vi "test TCX read (installed 71).vi"() -> ()   [LabVIEW 2011] (continued)
armin.com/xmlschemas/ActivityExtension/v2\"><Watts>297</Watts></TPX></Extensions></Trackpoint><Trackpoint><Time>2008-03-03T13:51:13Z</Time><Position><LatitudeDegrees>35.881028</LatitudeDegrees><LongitudeDegrees>-78.947664</LongitudeDegrees></Position><AltitudeMeters>84.733</AltitudeMeters><DistanceMeters>1639.767</DistanceMeters><Cadence>88</Cadence><Extensions><TPX xmlns=\"http://www.garmin.com/xmlschemas/ActivityExtension/v2\"><Watts>240</Watts></TPX></Extensions></Trackpoint><Trackpoint><Time>2008-03-03T13:51:14Z</Time><Position><LatitudeDegrees>35.880933</LatitudeDegrees><LongitudeDegrees>-78.947691</LongitudeDegrees></Position><AltitudeMeters>84.733</AltitudeMeters><DistanceMeters>1650.482</DistanceMeters><Cadence>88</Cadence><Extensions><TPX xmlns=\"http://www.garmin.com/xmlschemas/ActivityExtension/v2\"><Watts>161</Watts></TPX></Extensions></Trackpoint><Trackpoint><Time>2008-03-03T13:51:15Z</Time><Position><LatitudeDegrees>35.880839</LatitudeDegrees><LongitudeDegrees>-78.947718</LongitudeDegrees></Position><AltitudeMeters>84.733</AltitudeMeters><DistanceMeters>1661.201</DistanceMeters><Cadence>87</Cadence><Extensions><TPX xmlns=\"http://www.garmin.com/xmlschemas/ActivityExtension/v2\"><Watts>138</Watts></TPX></Extensions></Trackpoint><Trackpoint><Time>2008-03-03T13:51:16Z</Time><Position><LatitudeDegrees>35.880745</LatitudeDegrees><LongitudeDegrees>-78.947745</LongitudeDegrees></Position><AltitudeMeters>84.253</AltitudeMeters><DistanceMeters>1671.990</DistanceMeters><Cadence>88</Cadence><Extensions><TPX xmlns=\"http://www.garmin.com/xmlschemas/ActivityExtension/v2\"><Watts>130</Watts></TPX></Extensions></Trackpoint><Trackpoint><Time>2008-03-03T13:51:17Z</Time><Position><LatitudeDegrees>35.880651</LatitudeDegrees><LongitudeDegrees>-78.947772</LongitudeDegrees></Position><AltitudeMeters>84.253</AltitudeMeters><DistanceMeters>1682.650</DistanceMeters><Cadence>88</Cadence><Extensions><TPX xmlns=\"http://www.garmin.com/xmlschemas/ActivityExtension/v2\"><Watts>130</Watts></TPX></Extensions></Trackpoint><Trackpoint><Time>2008-03-03T13:51:18Z</Time><Position><LatitudeDegrees>35.880555</LatitudeDegrees><LongitudeDegrees>-78.947798</LongitudeDegrees></Position><AltitudeMeters>83.772</AltitudeMeters><DistanceMeters>1693.542</DistanceMeters><Cadence>89</Cadence><Extensions><TPX xmlns=\"http://www.garmin.com/xmlschemas/ActivityExtension/v2\"><Watts>138</Watts></TPX></Extensions></Trackpoint><Trackpoint><Time>2008-03-03T13:51:19Z</Time><Position><LatitudeDegrees>35.880459</LatitudeDegrees><LongitudeDegrees>-78.947824</LongitudeDegrees></Position><AltitudeMeters>83.772</AltitudeMeters><DistanceMeters>1704.492</DistanceMeters><Cadence>90</Cadence><Extensions><TPX xmlns=\"http://www.garmin.com/xmlschemas/ActivityExtension/v2\"><Watts>159</Watts></TPX></Extensions></Trackpoint><Trackpoint><Time>2008-03-03T13:51:20Z</Time><Position><LatitudeDegrees>35.880357</LatitudeDegrees><LongitudeDegrees>-78.947852</LongitudeDegrees></Position><AltitudeMeters>83.291</AltitudeMeters><DistanceMeters>1716.066</DistanceMeters><Cadence>90</Cadence><Extensions><TPX xmlns=\"http://www.garmin.com/xmlschemas/ActivityExtension/v2\"><Watts>168</Watts></TPX></Extensions></Trackpoint><Trackpoint><Time>2008-03-03T13:51:21Z</Time><Position><LatitudeDegrees>35.880258</LatitudeDegrees><LongitudeDegrees>-78.947880</LongitudeDegrees></Position><AltitudeMeters>82.811</AltitudeMeters><DistanceMeters>1727.394</DistanceMeters><Cadence>91</Cadence><Extensions><TPX xmlns=\"http://www.garmin.com/xmlschemas/ActivityExtension/v2\"><Watts>169</Watts></TPX></Extensions></Trackpoint><Trackpoint><Time>2008-03-03T13:51:22Z</Time><Position><LatitudeDegrees>35.880159</LatitudeDegrees><LongitudeDegrees>-78.947909</LongitudeDegrees></Position><AltitudeMeters>83.291</AltitudeMeters><DistanceMeters>1738.638</DistanceMeters><Cadence>90</Cadence><Extensions><TPX xmlns=\"http://www.garmin.com/xmlschemas/ActivityExtension/v2\"><Watts>163</Watts></TPX></Extensions></Trackpoint><Trackpoint><Time>2008-03-03T13:51:23Z</Time><Position><LatitudeDegrees>35.880061</LatitudeDegrees><LongitudeDegrees>-78.947936</LongitudeDegrees></Position><AltitudeMeters>82.811</AltitudeMeters><DistanceMeters>1749.873</DistanceMeters><Cadence>85</Cadence><Extensions><TPX xmlns=\"http://www.garmin.com/xmlschemas/ActivityExtension/v2\"><Watts>162</Watts></TPX></Extensions></Trackpoint><Trackpoint><Time>2008-03-03T13:51:24Z</Time><Position><LatitudeDegrees>35.879962</LatitudeDegrees><LongitudeDegrees>-78.947964</LongitudeDegrees></Position><AltitudeMeters>82.811</AltitudeMeters><DistanceMeters>1761.036</DistanceMeters><Cadence>85</Cadence><Extensions><TPX xmlns=\"http://www.garmin.com/xmlschemas/ActivityExtension/v2\"><Watts>162</Watts></TPX></Extensions></Trackpoint><Trackpoint><Time>2008-03-03T13:51:25Z</Time><Position><LatitudeDegrees>35.879864</LatitudeDegrees><LongitudeDegrees>-78.947991</LongitudeDegrees></Position><AltitudeMeters>82.330</AltitudeMeters><DistanceMeters>1772.261</DistanceMeters><Cadence>87</Cadence><Extensions><TPX xmlns=\"http://www.garmin.com/xmlschemas/ActivityExtension/v2\"><Watts>298</Watts></TPX></Extensions></Trackpoint><Trackpoint><Time>2008-03-03T13:51:26Z</Time><Position><LatitudeDegrees>35.879765</LatitudeDegrees><LongitudeDegrees>-78.948017</LongitudeDegrees></Position><AltitudeMeters>82.330</AltitudeMeters><DistanceMeters>1783.429</DistanceMeters><Cadence>87</Cadence><Extensions><TPX xmlns=\"http://www.garmin.com/xmlschemas/ActivityExtension/v2\"><Watts>301</Watts></TPX></Extensions></Trackpoint><Trackpoint><Time>2008-03-03T13:51:27Z</Time><Position><LatitudeDegrees>35.879669</LatitudeDegrees><LongitudeDegrees>-78.948046</LongitudeDegrees></Position><AltitudeMeters>81.849</AltitudeMeters><DistanceMeters>1794.441</DistanceMeters><Cadence>87</Cadence><Extensions><TPX xmlns=\"http://www.garmin.com/xmlschemas/ActivityExtension/v2\"><Watts>261</Watts></TPX></Extensions></Trackpoint><Trackpoint><Time>2008-03-03T13:51:28Z</Time><Position><LatitudeDegrees>35.879570</LatitudeDegrees><LongitudeDegrees>-78.948074</LongitudeDegrees></Position><AltitudeMeters>81.849</AltitudeMeters><DistanceMeters>1805.737</DistanceMeters><Cadence>88</Cadence><Extensions><TPX xmlns=\"http://www.garmin.com/xmlschemas/ActivityExtension/v2\"><Watts>224</Watts></TPX></Extensions></Trackpoint><Trackpoint><Time>2008-03-03T13:51:29Z</Time><Position><LatitudeDegrees>35.879469</LatitudeDegrees><LongitudeDegrees>-78.948102</LongitudeDegrees></Position><AltitudeMeters>81.369</AltitudeMeters><DistanceMeters>1817.204</DistanceMeters><Cadence>88</Cadence><Extensions><TPX xmlns=\"http://www.garmin.com/xmlschemas/ActivityExtension/v2\"><Watts>225</Watts></TPX></Extensions></Trackpoint><Trackpoint><Time>2008-03-03T13:51:30Z</Time><Position><LatitudeDegrees>35.879367</LatitudeDegrees><LongitudeDegrees>-78.948129</LongitudeDegrees></Position><AltitudeMeters>81.369</AltitudeMeters><DistanceMeters>1828.736</DistanceMeters><Cadence>86</Cadence><Extensions><TPX xmlns=\"http://www.garmin.com/xmlschemas/ActivityExtension/v2\"><Watts>204</Watts></TPX></Extensions></Trackpoint><Trackpoint><Time>2008-03-03T13:51:31Z</Time><Position><LatitudeDegrees>35.879267</LatitudeDegrees><LongitudeDegrees>-78.948157</LongitudeDegrees></Position><AltitudeMeters>81.369</AltitudeMeters><DistanceMeters>1840.158</DistanceMeters><Cadence>87</Cadence><Extensions><TPX xmlns=\"http://www.garmin.com/xmlschemas/ActivityExtension/v2\"><Watts>241</Watts></TPX></Extensions></Trackpoint><Trackpoint><Time>2008-03-03T13:51:32Z</Time><Position><LatitudeDegrees>35.879166</LatitudeDegrees><LongitudeDegrees>-78.948183</LongitudeDegrees></Position><AltitudeMeters>81.369</AltitudeMeters><DistanceMeters>1851.623</DistanceMeters><Cadence>87</Cadence><Extensions><TPX xmlns=\"http://www.garmin.com/xmlschemas/ActivityExtension/v2\"><Watts>287</Watts></TPX></Extensions></Trackpoint><Trackpoint><Time>2008-03-03T13:51:33Z</Time><Position><LatitudeDegrees>35.879065</LatitudeDegrees><LongitudeDegrees>-78.948209</LongitudeDegrees></Position><AltitudeMeters>80.888</AltitudeMeters><DistanceMeters>1863.054</DistanceMeters><Cadence>87</Cadence><Extensions><TPX xmlns=\"http://www.garmin.com/xmlschemas/ActivityExtension/v2\"><Watts>287</Watts></TPX></Extensions></Trackpoint><Trackpoint><Time>2008-03-03T13:51:34Z</Time><Position><LatitudeDegrees>35.878963</LatitudeDegrees><LongitudeDegrees>-78.948236</LongitudeDegrees></Position><AltitudeMeters>80.888</AltitudeMeters><DistanceMeters>1874.573</DistanceMeters><Cadence>0</Cadence></Trackpoint><Trackpoint><Time>2008-03-03T13:51:35Z</Time><Position><LatitudeDegrees>35.878863</LatitudeDegrees><LongitudeDegrees>-78.948263</LongitudeDegrees></Position><AltitudeMeters>80.888</AltitudeMeters><DistanceMeters>1885.957</DistanceMeters><Cadence>86</Cadence><Extensions><TPX xmlns=\"http://www.garmin.com/xmlschemas/ActivityExtension/v2\"><Watts>275</Watts></TPX></Extensions></Trackpoint><Trackpoint><Time>2008-03-03T13:51:36Z</Time><Position><LatitudeDegrees>35.878769</LatitudeDegrees><LongitudeDegrees>-78.948289</LongitudeDegrees></Position><AltitudeMeters>80.888</AltitudeMeters><DistanceMeters>1896.548</DistanceMeters><Cadence>86</Cadence><Extensions><TPX xmlns=\"http://www.garmin.com/xmlschemas/ActivityExtension/v2\"><Watts>275</Watts></TPX></Extensions></Trackpoint><Trackpoint><Time>2008-03-03T13:51:37Z</Time><Position><LatitudeDegrees>35.878677</LatitudeDegrees><LongitudeDegrees>-78.948315</LongitudeDegrees></Position><AltitudeMeters>80.888</AltitudeMeters><DistanceMeters>1907.055</DistanceMeters><Cadence>83</Cadence><Extensions><TPX xmlns=\"http://www.garmin.com/xmlschemas/ActivityExtension/v2\"><Watts>198</Watts></TPX></Extensions></Trackpoint><Trackpoint><Time>2008-03-03T13:51:38Z</Time><Position><LatitudeDegrees>35.878584</LatitudeDegrees><LongitudeDegrees>-78.948340</LongitudeDegrees></Position><AltitudeMeters>80.888</AltitudeMeters><DistanceMeters>1917.727</DistanceMeters><Cadence>82</Cadence><Extensions><TPX xmlns=\"http://www.garmin.com/xmlschemas/ActivityExtension/v2\"><Watts>193</Watts></TPX></Extensions></Trackpoint><Trackpoint><Time>2008-03-03T13:51:39Z</Time><Position><LatitudeDegrees>35.878491</LatitudeDegrees><LongitudeDegrees>-78.948363</LongitudeDegrees></Position><AltitudeMeters>80.888</AltitudeMeters><DistanceMeters>1928.120</DistanceMeters><Cadence>81</Cadence><Extensions><TPX xmlns=\"http://www.garmin.com/xmlschemas/ActivityExtension/v2\"><Watts>189</Watts></TPX></Extensions></Trackpoint><Trackpoint><Time>2008-03-03T13:51:40Z</Time><Position><LatitudeDegrees>35.878400</LatitudeDegrees><LongitudeDegrees>-78.948387</LongitudeDegrees></Position><AltitudeMeters>80.888</AltitudeMeters><DistanceMeters>1938.520</DistanceMeters><Cadence>79</Cadence><Extensions><TPX xmlns=\"http://www.garmin.com/xmlschemas/ActivityExtension/v2\"><Watts>206</Watts></TPX></Extensions></Trackpoint><Trackpoint><Time>2008-03-03T13:51:41Z</Time><Position><LatitudeDegrees>35.878309</LatitudeDegrees><LongitudeDegrees>-78.948411</LongitudeDegrees></Position><AltitudeMeters>80.888</AltitudeMeters><DistanceMeters>1948.745</DistanceMeters><Cadence>78</Cadence><Extensions><TPX xmlns=\"http://www.garmin.com/xmlschemas/ActivityExtension/v2\"><Watts>223</Watts></TPX></Extensions></Trackpoint><Trackpoint><Time>2008-03-03T13:51:42Z</Time><Position><LatitudeDegrees>35.878220</LatitudeDegrees><LongitudeDegrees>-78.948434</LongitudeDegrees></Position><AltitudeMeters>81.369</AltitudeMeters><DistanceMeters>1958.824</DistanceMeters><Cadence>76</Cadence><Extensions><TPX xmlns=\"http://www.garmin.com/xmlschemas/ActivityExtension/v2\"><Watts>215</Watts></TPX></Extensions></Trackpoint><Trackpoint><Time>2008-03-03T13:51:43Z</Time><Position><LatitudeDegrees>35.878133</LatitudeDegrees><LongitudeDegrees>-78.948457</LongitudeDegrees></Position><AltitudeMeters>81.369</AltitudeMeters><DistanceMeters>1968.813</DistanceMeters><Cadence>76</Cadence><Extensions><TPX xmlns=\"http://www.garmin.com/xmlschemas/ActivityExtension/v2\"><Watts>235</Watts></TPX></Extensions></Trackpoint><Trackpoint><Time>2008-03-03T13:51:44Z</Time><Position><LatitudeDegrees>35.878045</LatitudeDegrees><LongitudeDegrees>-78.948478</LongitudeDegrees></Position><AltitudeMeters>81.369</AltitudeMeters><DistanceMeters>1978.745</DistanceMeters><Cadence>75</Cadence><Extensions><TPX xmlns=\"http://www.garmin.com/xmlschemas/ActivityExtension/v2\"><Watts>258</Watts></TPX></Extensions></Trackpoint><Trackpoint><Time>2008-03-03T13:51:45Z</Time><Position><LatitudeDegrees>35.877959</LatitudeDegrees><LongitudeDegrees>-78.948499</LongitudeDegrees></Position><AltitudeMeters>81.369</AltitudeMeters><DistanceMeters>1988.499</DistanceMeters><Cadence>75</Cadence><Extensions><TPX xmlns=\"http://www.garmin.com/xmlschemas/ActivityExtension/v2\"><Watts>275</Watts></TPX></Extensions></Trackpoint><Trackpoint><Time>2008-03-03T13:51:46Z</Time><Position><LatitudeDegrees>35.877872</LatitudeDegrees><LongitudeDegrees>-78.948520</LongitudeDegrees></Position><AltitudeMeters>81.369</AltitudeMeters><DistanceMeters>1998.246</DistanceMeters><Cadence>75</Cadence><Extensions><TPX xmlns=\"http://www.garmin.com/xmlschemas/ActivityExtension/v2\"><Watts>276</Watts></TPX></Extensions></Trackpoint><Trackpoint><Time>2008-03-03T13:51:47Z</Time><Position><LatitudeDegrees>35.877787</LatitudeDegrees><LongitudeDegrees>-78.948541</LongitudeDegrees></Position><AltitudeMeters>81.369</AltitudeMeters><DistanceMeters>2007.902</DistanceMeters><Cadence>73</Cadence><Extensions><TPX xmlns=\"http://www.garmin.com/xmlschemas/ActivityExtension/v2\"><Watts>272</Watts></TPX></Extensions></Trackpoint><Trackpoint><Time>2008-03-03T13:51:48Z</Time><Position><LatitudeDegrees>35.877702</LatitudeDegrees><LongitudeDegrees>-78.948562</LongitudeDegrees></Position><AltitudeMeters>81.369</AltitudeMeters><DistanceMeters>2017.490</DistanceMeters><Cadence>73</Cadence><Extensions><TPX xmlns=\"http://www.garmin.com/xmlschemas/ActivityExtension/v2\"><Watts>271</Watts></TPX></Extensions></Trackpoint><Trackpoint><Time>2008-03-03T13:51:49Z</Time><Position><LatitudeDegrees>35.877619</LatitudeDegrees><LongitudeDegrees>-78.948581</LongitudeDegrees></Position><AltitudeMeters>81.369</AltitudeMeters><DistanceMeters>2026.826</DistanceMeters><Cadence>73</Cadence><Extensions><TPX xmlns=\"http://www.garmin.com/xmlschemas/ActivityExtension/v2\"><Watts>261</Watts></TPX></Extensions></Trackpoint><Trackpoint><Time>2008-03-03T13:51:50Z</Time><Position><LatitudeDegrees>35.877538</LatitudeDegrees><LongitudeDegrees>-78.948599</LongitudeDegrees></Position><AltitudeMeters>81.369</AltitudeMeters><DistanceMeters>2035.975</DistanceMeters><Cadence>72</Cadence><Extensions><TPX xmlns=\"http://www.garmin.com/xmlschemas/ActivityExtension/v2\"><Watts>250</Watts></TPX></Extensions></Trackpoint><Trackpoint><Time>2008-03-03T13:51:51Z</Time><Position><LatitudeDegrees>35.877456</LatitudeDegrees><LongitudeDegrees>-78.948620</LongitudeDegrees></Position><AltitudeMeters>81.849</AltitudeMeters><DistanceMeters>2045.245</DistanceMeters><Cadence>72</Cadence><Extensions><TPX xmlns=\"http://www.garmin.com/xmlschemas/ActivityExtension/v2\"><Watts>255</Watts></TPX></Extensions></Trackpoint><Trackpoint><Time>2008-03-03T13:51:52Z</Time><Position><LatitudeDegrees>35.877377</LatitudeDegrees><LongitudeDegrees>-78.948641</LongitudeDegrees></Position><AltitudeMeters>81.369</AltitudeMeters><DistanceMeters>2054.220</DistanceMeters><Cadence>71</Cadence><Extensions><TPX xmlns=\"http://www.garmin.com/xmlschemas/ActivityExtension/v2\"><Watts>255</Watts></TPX></Extensions></Trackpoint><Trackpoint><Time>2008-03-03T13:51:53Z</Time><Position><LatitudeDegrees>35.877302</LatitudeDegrees><LongitudeDegrees>-78.948661</LongitudeDegrees></Position><AltitudeMeters>81.849</AltitudeMeters><DistanceMeters>2062.803</DistanceMeters><Cadence>71</Cadence><Extensions><TPX xmlns=\"http://www.garmin.com/xmlschemas/ActivityExtension/v2\"><Watts>251</Watts></TPX></Extensions></Trackpoint><Trackpoint><Time>2008-03-03T13:51:54Z</Time><Position><LatitudeDegrees>35.877222</LatitudeDegrees><LongitudeDegrees>-78.948680</LongitudeDegrees></Position><AltitudeMeters>81.849</AltitudeMeters><DistanceMeters>2071.717</DistanceMeters><Cadence>71</Cadence><Extensions><TPX xmlns=\"http://www.garmin.com/xmlschemas/ActivityExtension/v2\"><Watts>251</Watts></TPX></Extensions></Trackpoint><Trackpoint><Time>2008-03-03T13:51:55Z</Time><Position><LatitudeDegrees>35.877150</LatitudeDegrees><LongitudeDegrees>-78.948701</LongitudeDegrees></Position><AltitudeMeters>82.330</AltitudeMeters><DistanceMeters>2079.870</DistanceMeters><Cadence>69</Cadence><Extensions><TPX xmlns=\"http://www.garmin.com/xmlschemas/ActivityExtension/v2\"><Watts>203</Watts></TPX></Extensions></Trackpoint><Trackpoint><Time>2008-03-03T13:51:56Z</Time><Position><LatitudeDegrees>35.877076</LatitudeDegrees><LongitudeDegrees>-78.948721</LongitudeDegrees></Position><AltitudeMeters>81.849</AltitudeMeters><DistanceMeters>2088.349</DistanceMeters><Cadence>69</Cadence><Extensions><TPX xmlns=\"http://www.garmin.com/xmlschemas/ActivityExtension/v2\"><Watts>204</Watts></TPX></Extensions></Trackpoint><Trackpoint><Time>2008-03-03T13:51:57Z</Time><Position><LatitudeDegrees>35.877000</LatitudeDegrees><LongitudeDegrees>-78.948743</LongitudeDegrees></Position><AltitudeMeters>82.330</AltitudeMeters><DistanceMeters>2097.061</DistanceMeters><Cadence>69</Cadence><Extensions><TPX xmlns=\"http://www.garmin.com/xmlschemas/ActivityExtension/v2\"><Watts>231</Watts></TPX></Extensions></Trackpoint><Trackpoint><Time>2008-03-03T13:51:58Z</Time><Position><LatitudeDegrees>35.876922</LatitudeDegrees><LongitudeDegrees>-78.948765</LongitudeDegrees></Position><AltitudeMeters>82.811</AltitudeMeters><DistanceMeters>2105.914</DistanceMeters><Cadence>69</Cadence><Extensions><TPX xmlns=\"http://www.garmin.com/xmlschemas/ActivityExtension/v2\"><Watts>262</Watts></TPX></Extensions></Trackpoint><Trackpoint><Time>2008-03-03T13:51:59Z</Time><Position><LatitudeDegrees>35.876846</LatitudeDegrees><LongitudeDegrees>-78.948789</LongitudeDegrees></Position><AltitudeMeters>82.330</AltitudeMeters><DistanceMeters>2114.597</DistanceMeters><Cadence>68</Cadence><Extensions><TPX xmlns=\"http://www.garmin.com/xmlschemas/ActivityExtension/v2\"><Watts>272</Watts></TPX></Extensions></Trackpoint><Trackpoint><Time>2008-03-03T13:52:00Z</Time><Position><LatitudeDegrees>35.876770</LatitudeDegrees><LongitudeDegrees>-78.948813</LongitudeDegrees></Position><AltitudeMeters>82.811</AltitudeMeters><DistanceMeters>2123.349</DistanceMeters><Cadence>68</Cadence><Extensions><TPX xmlns=\"http://www.garmin.com/xmlschemas/ActivityExtension/v2\"><Watts>274</Watts></TPX></Extensions></Trackpoint><Trackpoint><Time>2008-03-03T13:52:01Z</Time><Position><LatitudeDegrees>35.876696</LatitudeDegrees><LongitudeDegrees>-78.948837</LongitudeDegrees></Position><AltitudeMeters>82.330</AltitudeMeters><DistanceMeters>2131.821</DistanceMeters><Cadence>68</Cadence><Extensions><TPX xmlns=\"http://www.garmin.com/xmlschemas/ActivityExtension/v2\"><Watts>272</Watts></TPX></Extensions></Trackpoint><Trackpoint><Time>2008-03-03T13:52:02Z</Time><Position><LatitudeDegrees>35.876620</LatitudeDegrees><LongitudeDegrees>-78.948857</LongitudeDegrees></Position><AltitudeMeters>82.811</AltitudeMeters><DistanceMeters>2140.467</DistanceMeters><Cadence>66</Cadence><Extensions><TPX xmlns=\"http://www.garmin.com/xmlschemas/ActivityExtension/v2\"><Watts>234</Watts></TPX></Extensions></Trackpoint><Trackpoint><Time>2008-03-03T13:52:03Z</Time><Position><LatitudeDegrees>35.876545</LatitudeDegrees><LongitudeDegrees>-78.948874</LongitudeDegrees></Position><AltitudeMeters>82.811</AltitudeMeters><DistanceMeters>2148.926</DistanceMeters><Cadence>64</Cadence><Extensions><TPX xmlns=\"http://www.garmin.com/xmlschemas/ActivityExtension/v2\"><Watts>203</Watts></TPX></Extensions></Trackpoint><Trackpoint><Time>2008-03-03T13:52:04Z</Time><Position><LatitudeDegrees>35.876479</LatitudeDegrees><LongitudeDegrees>-78.948891</LongitudeDegrees></Position><AltitudeMeters>82.811</AltitudeMeters><DistanceMeters>2156.350</DistanceMeters><Cadence>64</Cadence><Extensions><TPX xmlns=\"http://www.garmin.com/xmlschemas/ActivityExtension/v2\"><Watts>202</Watts></TPX></Extensions></Trackpoint><Trackpoint><Time>2008-03-03T13:52:05Z</Time><Position><LatitudeDegrees>35.876410</LatitudeDegrees><LongitudeDegrees>-78.948902</LongitudeDegrees></Position><AltitudeMeters>83.291</AltitudeMeters><DistanceMeters>2164.018</DistanceMeters><Cadence>61</Cadence><Extensions><TPX xmlns=\"http://www.garmin.com/xmlschemas/ActivityExtension/v2\"><Watts>174</Watts></TPX></Extensions></Trackpoint><Trackpoint><Time>2008-03-03T13:52:06Z</Time><Position><LatitudeDegrees>35.876346</LatitudeDegrees><LongitudeDegrees>-78.948895</LongitudeDegrees></Position><AltitudeMeters>83.772</AltitudeMeters><DistanceMeters>2171.119</DistanceMeters><Cadence>61</Cadence><Extensions><TPX xmlns=\"http://www.garmin.com/xmlschemas/ActivityExtension/v2\"><Watts>172</Watts></TPX></Extensions></Trackpoint><Trackpoint><Time>2008-03-03T13:52:07Z</Time><Position><LatitudeDegrees>35.876286</LatitudeDegrees><LongitudeDegrees>-78.948858</LongitudeDegrees></Position><AltitudeMeters>83.772</AltitudeMeters><DistanceMeters>2178.391</DistanceMeters><Cadence>59</Cadence><Extensions><TPX xmlns=\"http://www.garmin.com/xmlschemas/ActivityExtension/v2\"><Watts>182</Watts></TPX></Extensions></Trackpoint><Trackpoint><Time>2008-03-03T13:52:08Z</Time><Position><LatitudeDegrees>35.876241</LatitudeDegrees><LongitudeDegrees>-78.948796</LongitudeDegrees></Position><AltitudeMeters>83.291</AltitudeMeters><DistanceMeters>2186.050</DistanceMeters><Cadence>58</Cadence><Extensions><TPX xmlns=\"http://www.garmin.com/xmlschemas/ActivityExtension/v2\"><Watts>161</Watts></TPX></Extensions></Trackpoint><Trackpoint><Time>2008-03-03T13:52:09Z</Time><Position><LatitudeDegrees>35.876209</LatitudeDegrees><LongitudeDegrees>-78.948716</LongitudeDegrees></Position><AltitudeMeters>83.291</AltitudeMeters><DistanceMeters>2194.065</DistanceMeters><Cadence>60</Cadence><Extensions><TPX xmlns=\"http://www.garmin.com/xmlschemas/ActivityExtension/v2\"><Watts>170</Watts></TPX></Extensions></Trackpoint><Trackpoint><Time>2008-03-03T13:52:10Z</Time><Position><LatitudeDegrees>35.876192</LatitudeDegrees><LongitudeDegrees>-78.948626</LongitudeDegrees></Position><AltitudeMeters>83.291</AltitudeMeters><DistanceMeters>2202.401</DistanceMeters><Cadence>61</Cadence><Extensions><TPX xmlns=\"http://www.garmin.com/xmlschemas/ActivityExtension/v2\"><Watts>168</Watts></TPX></Extensions></Trackpoint><Trackpoint><Time>2008-03-03T13:52:11Z</Time><Position><LatitudeDegrees>35.876196</LatitudeDegrees><LongitudeDegrees>-78.948531</LongitudeDegrees></Position><AltitudeMeters>83.291</AltitudeMeters><DistanceMeters>2210.917</DistanceMeters><Cadence>61</Cadence><Extensions><TPX xmlns=\"http://www.garmin.com/xmlschemas/ActivityExtension/v2\"><Watts>169</Watts></TPX></Extensions></Trackpoint><Trackpoint><Time>2008-03-03T13:52:12Z</Time><Position><LatitudeDegrees>35.876189</LatitudeDegrees><LongitudeDegrees>-78.948433</LongitudeDegrees></Position><AltitudeMeters>83.291</AltitudeMeters><DistanceMeters>2219.879</DistanceMeters><Cadence>66</Cadence><Extensions><TPX xmlns=\"http://www.garmin.com/xmlschemas/ActivityExtension/v2\"><Watts>212</Watts></TPX></Extensions></Trackpoint><Trackpoint><Time>2008-03-03T13:52:13Z</Time><Position><LatitudeDegrees>35.876186</LatitudeDegrees><LongitudeDegrees>-78.948331</LongitudeDegrees></Position><AltitudeMeters>82.811</AltitudeMeters><DistanceMeters>2229.032</DistanceMeters><Cadence>66</Cadence><Extensions><TPX xmlns=\"http://www.garmin.com/xmlschemas/ActivityExtension/v2\"><Watts>213</Watts></TPX></Extensions></Trackpoint><Trackpoint><Time>2008-03-03T13:52:14Z</Time><Position><LatitudeDegrees>35.876190</LatitudeDegrees><LongitudeDegrees>-78.948228</LongitudeDegrees></Position><AltitudeMeters>82.330</AltitudeMeters><DistanceMeters>2238.333</DistanceMeters><Cadence>71</Cadence><Extensions><TPX xmlns=\"http://www.garmin.com/xmlschemas/ActivityExtension/v2\"><Watts>193</Watts></TPX></Extensions></Trackpoint><Trackpoint><Time>2008-03-03T13:52:15Z</Time><Position><LatitudeDegrees>35.876188</LatitudeDegrees><LongitudeDegrees>-78.948122</LongitudeDegrees></Position><AltitudeMeters>82.811</AltitudeMeters><DistanceMeters>2247.949</DistanceMeters><Cadence>72</Cadence><Extensions><TPX xmlns=\"http://www.garmin.com/xmlschemas/ActivityExtension/v2\"><Watts>174</Watts></TPX></Extensions></Trackpoint><Trackpoint><Time>2008-03-03T13:52:16Z</Time><Position><LatitudeDegrees>35.876189</LatitudeDegrees><LongitudeDegrees>-78.948014</LongitudeDegrees></Position><AltitudeMeters>82.330</AltitudeMeters><DistanceMeters>2257.651</DistanceMeters><Cadence>72</Cadence><Extensions><TPX xmlns=\"http://www.garmin.com/xmlschemas/ActivityExtension/v2\"><Watts>174</Watts></TPX></Extensions></Trackpoint><Trackpoint><Time>2008-03-03T13:52:17Z</Time><Position><LatitudeDegrees>35.876190</LatitudeDegrees><LongitudeDegrees>-78.947905</LongitudeDegrees></Position><AltitudeMeters>82.811</AltitudeMeters><DistanceMeters>2267.518</DistanceMeters><Cadence>74</Cadence><Extensions><TPX xmlns=\"http://www.garmin.com/xmlschemas/ActivityExtension/v2\"><Watts>162</Watts></TPX></Extensions></Trackpoint><Trackpoint><Time>2008-03-03T13:52:18Z</Time><Position><LatitudeDegrees>35.876186</LatitudeDegrees><LongitudeDegrees>-78.947794</LongitudeDegrees></Position><AltitudeMeters>81.849</AltitudeMeters><DistanceMeters>2277.555</DistanceMeters><Cadence>75</Cadence><Extensions><TPX xmlns=\"http://www.garmin.com/xmlschemas/ActivityExtension/v2\"><Watts>156</Watts></TPX></Extensions></Trackpoint><Trackpoint><Time>2008-03-03T13:52:19Z</Time><Position><LatitudeDegrees>35.876185</LatitudeDegrees><LongitudeDegrees>-78.947683</LongitudeDegrees></Position><AltitudeMeters>82.330</AltitudeMeters><DistanceMeters>2287.656</DistanceMeters><Cadence>76</Cadence><Extensions><TPX xmlns=\"http://www.garmin.com/xmlschemas/ActivityExtension/v2\"><Watts>171</Watts></TPX></Extensions></Trackpoint><Trackpoint><Time>2008-03-03T13:52:20Z</Time><Position><LatitudeDegrees>35.876184</LatitudeDegrees><LongitudeDegrees>-78.947570</LongitudeDegrees></Position><AltitudeMeters>81.369</AltitudeMeters><DistanceMeters>2297.795</DistanceMeters><Cadence>77</Cadence><Extensions><TPX xmlns=\"http://www.garmin.com/xmlschemas/ActivityExtension/v2\"><Watts>173</Watts></TPX></Extensions></Trackpoint><Trackpoint><Time>2008-03-03T13:52:21Z</Time><Position><LatitudeDegrees>35.876180</LatitudeDegrees><LongitudeDegrees>-78.947457</LongitudeDegrees></Position><AltitudeMeters>81.849</AltitudeMeters><DistanceMeters>2308.072</DistanceMeters><Cadence>77</Cadence><Extensions><TPX xmlns=\"http://www.garmin.com/xmlschemas/ActivityExtension/v2\"><Watts>160</Watts></TPX></Extensions></Trackpoint><Trackpoint><Time>2008-03-03T13:52:22Z</Time><Position><LatitudeDegrees>35.876177</LatitudeDegrees><LongitudeDegrees>-78.947343</LongitudeDegrees></Position><AltitudeMeters>80.888</AltitudeMeters><DistanceMeters>2318.399</DistanceMeters><Cadence>78</Cadence><Extensions><TPX xmlns=\"http://www.garmin.com/xmlschemas/ActivityExtension/v2\"><Watts>133</Watts></TPX></Extensions></Trackpoint><Trackpoint><Time>2008-03-03T13:52:23Z</Time><Position><LatitudeDegrees>35.876169</LatitudeDegrees><LongitudeDegrees>-78.947228</LongitudeDegrees></Position><AltitudeMeters>80.888</AltitudeMeters><DistanceMeters>2328.826</DistanceMeters><Cadence>78</Cadence><Extensions><TPX xmlns=\"http://www.garmin.com/xmlschemas/ActivityExtension/v2\"><Watts>132</Watts></TPX></Extensions></Trackpoint><Trackpoint><Time>2008-03-03T13:52:24Z</Time><Position><LatitudeDegrees>35.876157</LatitudeDegrees><LongitudeDegrees>-78.947112</LongitudeDegrees></Position><AltitudeMeters>80.407</AltitudeMeters><DistanceMeters>2339.331</DistanceMeters><Cadence>79</Cadence><Extensions><TPX xmlns=\"http://www.garmin.com/xmlschemas/ActivityExtension/v2\"><Watts>137</Watts></TPX></Extensions></Trackpoint><Trackpoint><Time>2008-03-03T13:52:25Z</Time><Position><LatitudeDegrees>35.876155</LatitudeDegrees><LongitudeDegrees>-78.946996</LongitudeDegrees></Position><AltitudeMeters>80.888</AltitudeMeters><DistanceMeters>2349.869</DistanceMeters><Cadence>80</Cadence><Extensions><TPX xmlns=\"http://www.garmin.com/xmlschemas/ActivityExtension/v2\"><Watts>136</Watts></TPX></Extensions></Trackpoint><Trackpoint><Time>2008-03-03T13:52:26Z</Time><Position><LatitudeDegrees>35.876153</LatitudeDegrees><LongitudeDegrees>-78.946876</LongitudeDegrees></Position><AltitudeMeters>79.927</AltitudeMeters><DistanceMeters>2360.659</DistanceMeters><Cadence>81</Cadence><Extensions><TPX xmlns=\"http://www.garmin.com/xmlschemas/ActivityExtension/v2\"><Watts>150</Watts></TPX></Extensions></Trackpoint><Trackpoint><Time>2008-03-03T13:52:27Z</Time><Position><LatitudeDegrees>35.876150</LatitudeDegrees><LongitudeDegrees>-78.946755</LongitudeDegrees></Position><AltitudeMeters>79.927</AltitudeMeters><DistanceMeters>2371.618</DistanceMeters><Cadence>82</Cadence><Extensions><TPX xmlns=\"http://www.garmin.com/xmlschemas/ActivityExtension/v2\"><Watts>153</Watts></TPX></Extensions></Trackpoint><Trackpoint><Time>2008-03-03T13:52:28Z</Time><Position><LatitudeDegrees>35.876150</LatitudeDegrees><LongitudeDegrees>-78.946632</LongitudeDegrees></Position><AltitudeMeters>79.446</AltitudeMeters><DistanceMeters>2382.706</DistanceMeters><Cadence>83</Cadence><Extensions><TPX xmlns=\"http://www.garmin.com/xmlschemas/ActivityExtension/v2\"><Watts>142</Watts></TPX></Extensions></Trackpoint><Trackpoint><Time>2008-03-03T13:52:29Z</Time><Position><LatitudeDegrees>35.876147</LatitudeDegrees><LongitudeDegrees>-78.946509</LongitudeDegrees></Position><AltitudeMeters>78.965</AltitudeMeters><DistanceMeters>2393.848</DistanceMeters><Cadence>84</Cadence><Extensions><TPX xmlns=\"http://www.garmin.com/xmlschemas/ActivityExtension/v2\"><Watts>125</Watts></TPX></Extensions></Trackpoint><Trackpoint><Time>2008-03-03T13:52:30Z</Time><Position><LatitudeDegrees>35.876144</LatitudeDegrees><LongitudeDegrees>-78.946385</LongitudeDegrees></Position><AltitudeMeters>78.485</AltitudeMeters><DistanceMeters>2405.011</DistanceMeters><Cadence>84</Cadence><Extensions><TPX xmlns=\"http://www.garmin.com/xmlschemas/ActivityExtension/v2\"><Watts>124</Watts></TPX></Extensions></Trackpoint><Trackpoint><Time>2008-03-03T13:52:31Z</Time><Position><LatitudeDegrees>35.876141</LatitudeDegrees><LongitudeDegrees>-78.946261</LongitudeDegrees></Position><AltitudeMeters>78.485</AltitudeMeters><DistanceMeters>2416.295</DistanceMeters><Cadence>84</Cadence><Extensions><TPX xmlns=\"http://www.garmin.com/xmlschemas/ActivityExtension/v2\"><Watts>122</Watts></TPX></Extensions></Trackpoint><Trackpoint><Time>2008-03-03T13:52:32Z</Time><Position><LatitudeDegrees>35.876138</LatitudeDegrees><LongitudeDegrees>-78.946136</LongitudeDegrees></Position><AltitudeMeters>78.004</AltitudeMeters><DistanceMeters>2427.554</DistanceMeters><Cadence>86</Cadence><Extensions><TPX xmlns=\"http://www.garmin.com/xmlschemas/ActivityExtension/v2\"><Watts>135</Watts></TPX></Extensions></Trackpoint><Trackpoint><Time>2008-03-03T13:52:33Z</Time><Position><LatitudeDegrees>35.876135</LatitudeDegrees><LongitudeDegrees>-78.946010</LongitudeDegrees></Position><AltitudeMeters>78.004</AltitudeMeters><DistanceMeters>2438.952</DistanceMeters><Cadence>87</Cadence><Extensions><TPX xmlns=\"http://www.garmin.com/xmlschemas/ActivityExtension/v2\"><Watts>142</Watts></TPX></Extensions></Trackpoint><Trackpoint><Time>2008-03-03T13:52:34Z</Time><Position><LatitudeDegrees>35.876134</LatitudeDegrees><LongitudeDegrees>-78.945881</LongitudeDegrees></Position><AltitudeMeters>78.004</AltitudeMeters><DistanceMeters>2450.581</DistanceMeters><Cadence>81</Cadence><Extensions><TPX xmlns=\"http://www.garmin.com/xmlschemas/ActivityExtension/v2\"><Watts>146</Watts></TPX></Extensions></Trackpoint><Trackpoint><Time>2008-03-03T13:52:35Z</Time><Position><LatitudeDegrees>35.876125</LatitudeDegrees><LongitudeDegrees>-78.945753</LongitudeDegrees></Position><AltitudeMeters>77.523</AltitudeMeters><DistanceMeters>2462.220</DistanceMeters><Cadence>81</Cadence><Extensions><TPX xmlns=\"http://www.garmin.com/xmlschemas/ActivityExtension/v2\"><Watts>150</Watts></TPX></Extensions></Trackpoint><Trackpoint><Time>2008-03-03T13:52:36Z</Time><Position><LatitudeDegrees>35.876118</LatitudeDegrees><LongitudeDegrees>-78.945623</LongitudeDegrees></Position><AltitudeMeters>77.523</AltitudeMeters><DistanceMeters>2473.962</DistanceMeters><Cadence>83</Cadence><Extensions><TPX xmlns=\"http://www.garmin.com/xmlschemas/ActivityExtension/v2\"><Watts>167</Watts></TPX></Extensions></Trackpoint><Trackpoint><Time>2008-03-03T13:52:37Z</Time><Position><LatitudeDegrees>35.876113</LatitudeDegrees><LongitudeDegrees>-78.945491</LongitudeDegrees></Position><AltitudeMeters>77.043</AltitudeMeters><DistanceMeters>2485.898</DistanceMeters><Cadence>84</Cadence><Extensions><TPX xmlns=\"http://www.garmin.com/xmlschemas/ActivityExtension/v2\"><Watts>180</Watts></TPX></Extensions></Trackpoint><Trackpoint><Time>2008-03-03T13:52:38Z</Time><Position><LatitudeDegrees>35.876110</LatitudeDegrees><LongitudeDegrees>-78.945358</LongitudeDegrees></Position><AltitudeMeters>76.562</AltitudeMeters><DistanceMeters>2497.959</DistanceMeters><Cadence>85</Cadence><Extensions><TPX xmlns=\"http://www.garmin.com/xmlschemas/ActivityExtension/v2\"><Watts>179</Watts></TPX></Extensions></Trackpoint><Trackpoint><Time>2008-03-03T13:52:39Z</Time><Position><LatitudeDegrees>35.876109</LatitudeDegrees><LongitudeDegrees>-78.945223</LongitudeDegrees></Position><AltitudeMeters>76.081</AltitudeMeters><DistanceMeters>2510.106</DistanceMeters><Cadence>85</Cadence><Extensions><TPX xmlns=\"http://www.garmin.com/xmlschemas/ActivityExtension/v2\"><Watts>202</Watts></TPX></Extensions></Trackpoint><Trackpoint><Time>2008-03-03T13:52:40Z</Time><Position><LatitudeDegrees>35.876106</LatitudeDegrees><LongitudeDegrees>-78.945087</LongitudeDegrees></Position><AltitudeMeters>75.601</AltitudeMeters><DistanceMeters>2522.354</DistanceMeters><Cadence>86</Cadence><Extensions><TPX xmlns=\"http://www.garmin.com/xmlschemas/ActivityExtension/v2\"><Watts>214</Watts></TPX></Extensions></Trackpoint><Trackpoint><Time>2008-03-03T13:52:41Z</Time><Position><LatitudeDegrees>35.876102</LatitudeDegrees><LongitudeDegrees>-78.944950</LongitudeDegrees></Position><AltitudeMeters>75.120</AltitudeMeters><DistanceMeters>2534.864</DistanceMeters><Cadence>87</Cadence><Extensions><TPX xmlns=\"http://www.garmin.com/xmlschemas/ActivityExtension/v2\"><Watts>206</Watts></TPX></Extensions></Trackpoint><Trackpoint><Time>2008-03-03T13:52:42Z</Time><Position><LatitudeDegrees>35.876098</LatitudeDegrees><LongitudeDegrees>-78.944811</LongitudeDegrees></Position><AltitudeMeters>75.120</AltitudeMeters><DistanceMeters>2547.381</DistanceMeters><Cadence>88</Cadence><Extensions><TPX xmlns=\"http://www.garmin.com/xmlschemas/ActivityExtension/v2\"><Watts>154</Watts></TPX></Extensions></Trackpoint><Trackpoint><Time>2008-03-03T13:52:43Z</Time><Position><LatitudeDegrees>35.876094</LatitudeDegrees><LongitudeDegrees>-78.944671</LongitudeDegrees></Position><AltitudeMeters>74.640</AltitudeMeters><DistanceMeters>2560.057</DistanceMeters><Cadence>88</Cadence><Extensions><TPX xmlns=\"http://www.garmin.com/xmlschemas/ActivityExtension/v2\"><Watts>162</Watts></TPX></Extensions></Trackpoint><Trackpoint><Time>2008-03-03T13:52:44Z</Time><Position><LatitudeDegrees>35.876089</LatitudeDegrees><LongitudeDegrees>-78.944530</LongitudeDegrees></Position><AltitudeMeters>73.678</AltitudeMeters><DistanceMeters>2572.833</DistanceMeters><Cadence>89</Cadence><Extensions><TPX xmlns=\"http://www.garmin.com/xmlschemas/ActivityExtension/v2\"><Watts>173</Watts></TPX></Extensions></Trackpoint><Trackpoint><Time>2008-03-03T13:52:45Z</Time><Position><LatitudeDegrees>35.876084</LatitudeDegrees><LongitudeDegrees>-78.944388</LongitudeDegrees></Position><AltitudeMeters>73.198</AltitudeMeters><DistanceMeters>2585.632</DistanceMeters><Cadence>89</Cadence><Extensions><TPX xmlns=\"http://www.garmin.com/xmlschemas/ActivityExtension/v2\"><Watts>174</Watts></TPX></Extensions></Trackpoint><Trackpoint><Time>2008-03-03T13:52:46Z</Time><Position><LatitudeDegrees>35.876081</LatitudeDegrees><LongitudeDegrees>-78.944245</LongitudeDegrees></Position><AltitudeMeters>73.198</AltitudeMeters><DistanceMeters>2598.556</DistanceMeters><Cadence>90</Cadence><Extensions><TPX xmlns=\"http://www.garmin.com/xmlschemas/ActivityExtension/v2\"><Watts>188</Watts></TPX></Extensions></Trackpoint><Trackpoint><Time>2008-03-03T13:52:47Z</Time><Position><LatitudeDegrees>35.876077</LatitudeDegrees><LongitudeDegrees>-78.944102</LongitudeDegrees></Position><AltitudeMeters>73.198</AltitudeMeters><DistanceMeters>2611.419</DistanceMeters><Cadence>90</Cadence><Extensions><TPX xmlns=\"http://www.garmin.com/xmlschemas/ActivityExtension/v2\"><Watts>182</Watts></TPX></Extensions></Trackpoint><Trackpoint><Time>2008-03-03T13:52:48Z</Time><Position><LatitudeDegrees>35.876074</LatitudeDegrees><LongitudeDegrees>-78.943960</LongitudeDegrees></Position><AltitudeMeters>72.717</AltitudeMeters><DistanceMeters>2624.305</DistanceMeters><Cadence>90</Cadence><Extensions><TPX xmlns=\"http://www.garmin.com/xmlschemas/ActivityExtension/v2\"><Watts>173</Watts></TPX></Extensions></Trackpoint><Trackpoint><Time>2008-03-03T13:52:49Z</Time><Position><LatitudeDegrees>35.876069</LatitudeDegrees><LongitudeDegrees>-78.943818</LongitudeDegrees></Position><AltitudeMeters>72.236</AltitudeMeters><DistanceMeters>2637.101</DistanceMeters><Cadence>90</Cadence><Extensions><TPX xmlns=\"http://www.garmin.com/xmlschemas/ActivityExtension/v2\"><Watts>174</Watts></TPX></Extensions></Trackpoint><Trackpoint><Time>2008-03-03T13:52:50Z</Time><Position><LatitudeDegrees>35.876065</LatitudeDegrees><LongitudeDegrees>-78.943677</LongitudeDegrees></Position><AltitudeMeters>71.755</AltitudeMeters><DistanceMeters>2649.851</DistanceMeters><Cadence>90</Cadence><Extensions><TPX xmlns=\"http://www.garmin.com/xmlschemas/ActivityExtension/v2\"><Watts>173</Watts></TPX></Extensions></Trackpoint><Trackpoint><Time>2008-03-03T13:52:51Z</Time><Position><LatitudeDegrees>35.876061</LatitudeDegrees><LongitudeDegrees>-78.943537</LongitudeDegrees></Position><AltitudeMeters>71.755</AltitudeMeters><DistanceMeters>2662.480</DistanceMeters><Cadence>88</Cadence><Extensions><TPX xmlns=\"http://www.garmin.com/xmlschemas/ActivityExtension/v2\"><Watts>171</Watts></TPX></Extensions></Trackpoint><Trackpoint><Time>2008-03-03T13:52:52Z</Time><Position><LatitudeDegrees>35.876054</LatitudeDegrees><LongitudeDegrees>-78.943398</LongitudeDegrees></Position><AltitudeMeters>71.755</AltitudeMeters><DistanceMeters>2675.059</DistanceMeters><Cadence>87</Cadence><Extensions><TPX xmlns=\"http://www.garmin.com/xmlschemas/ActivityExtension/v2\"><Watts>154</Watts></TPX></Extensions></Trackpoint><Trackpoint><Time>2008-03-03T13:52:53Z</Time><Position><LatitudeDegrees>35.876051</LatitudeDegrees><LongitudeDegrees>-78.943262</LongitudeDegrees></Position><AltitudeMeters>71.755</AltitudeMeters><DistanceMeters>2687.314</DistanceMeters><Cadence>87</Cadence><Extensions><TPX xmlns=\"http://www.garmin.com/xmlschemas/ActivityExtension/v2\"><Watts>155</Watts></TPX></Extensions></Trackpoint><Trackpoint><Time>2008-03-03T13:52:54Z</Time><Position><LatitudeDegrees>35.876049</LatitudeDegrees><LongitudeDegrees>-78.943130</LongitudeDegrees></Position><AltitudeMeters>71.755</AltitudeMeters><DistanceMeters>2699.239</DistanceMeters><Cadence>84</Cadence><Extensions><TPX xmlns=\"http://www.garmin.com/xmlschemas/ActivityExtension/v2\"><Watts>151</Watts></TPX></Extensions></Trackpoint><Trackpoint><Time>2008-03-03T13:52:55Z</Time><Position><LatitudeDegrees>35.876043</LatitudeDegrees><LongitudeDegrees>-78.942999</LongitudeDegrees></Position><AltitudeMeters>71.275</AltitudeMeters><DistanceMeters>2711.063</DistanceMeters><Cadence>83</Cadence><Extensions><TPX xmlns=\"http://www.garmin.com/xmlschemas/ActivityExtension/v2\"><Watts>1
